vi "Is Initialized.vi"(8 "Error In":errorcluster, 11 "reference in":refnum<class "Thermometer Multichannel.lvclass">) -> (0 "Error Out":errorcluster, 2 "Is Initialized?":bool, 3 "reference out":refnum<class "Thermometer Multichannel.lvclass">)   [LabVIEW 2024, in "Thermometer Multichannel.lvclass"]
uses:
  Thermometer Multichannel.lvclass
  Thermometer Multichannel.lvclass/Thermometer Multichannel.ctl
  Interfaces/IConfigure/IConfigure.lvclass
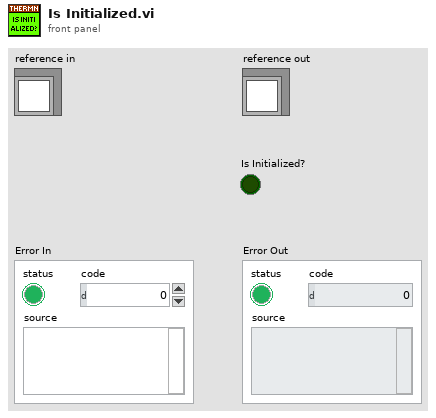
[diagram p1: front panel]
types:
  T1 = typedef "Thermometer Multichannel.lvclass/ObjectAttributes.ctl" = cluster{"IConfigure":refnum<class "IConfigure.lvclass">, "Worker Enqueuer":refnum<class "Message Enqueuer.lvclass">}
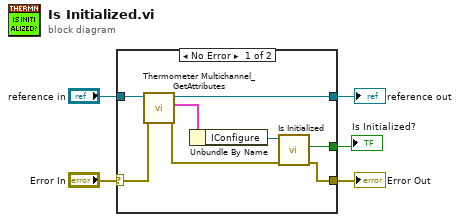
[diagram p0: block diagram]
diagram:
  n1 = case shown="No Error" "Error In" {
    selector: "Error In" -> [w13 w15]
    tunnel: [w6 w15] -> w4
    tunnel: [w10 w14] -> w2
    tunnel: "reference in" -> [w11 w14]
    tunnel: [w7 _] -> w1
    frame No Error {
      n2 = call "Thermometer Multichannel_GetAttributes.vi"("Error In"=w13, "reference in"=w11) -> ("Error Out"=w8:errorcluster, "Data"=w12:T1, "reference out"=w10:refnum<class "Thermometer Multichannel.lvclass">)  [unwired: 6 in, 1 out]
      n3 = Unbundle By Name(w12) -> ("IConfigure"=w9:refnum<class "IConfigure.lvclass">)
      n4 = call-dynamic "Is Initialized.vi"("error in"=w8, "IInitialize in"=w9) -> ("error out"=w6:errorcluster, "Is Initialized?"=w7:bool)  [unwired: 7 in, 1 out]
    }
    frame Error {
    }
  }
  "Error Out" <- w4
  "reference out" <- w2
  "Is Initialized?" <- w1
